vi "top level vi.vi"() -> ()   [LabVIEW 2014]
panel:
  in  "CtoF":bool
  out "Smallest":dbl
  out "greatest":dbl
  out "average value":dbl
  in  "WS":bool
  in  "stop":bool
  out "Waveform Chart":cluster{"random temp":dbl, dbl}(graph)
  # "(0~50 Celsius)"
  # "Summer"
  # "Winter"
  # "(-50~0 Celsius)"
  # "Fahrenheit"
  # "Celsius"
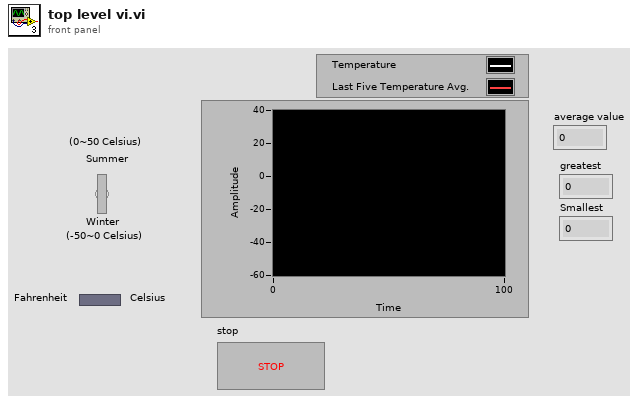
[diagram p1: front panel]
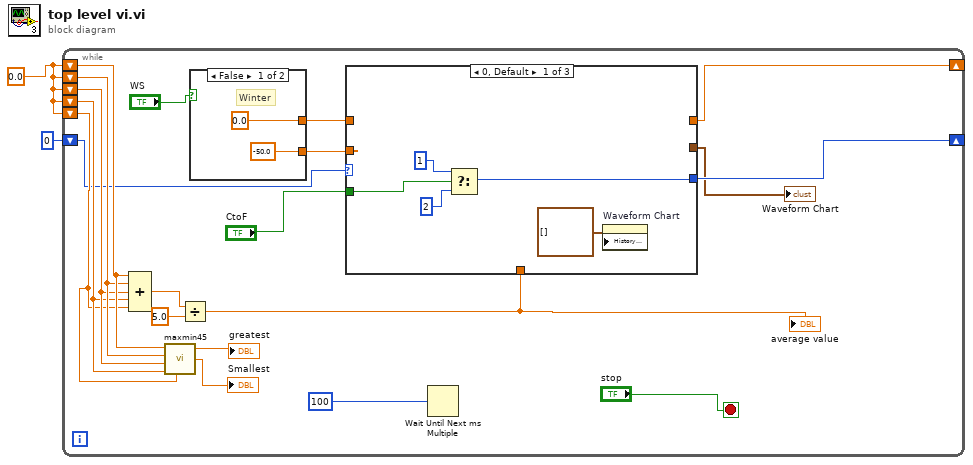
[diagram p0: block diagram]
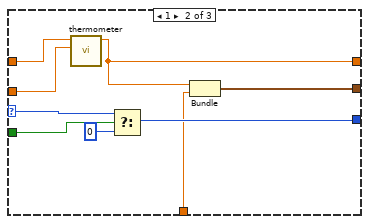
[diagram p2: hidden frame]
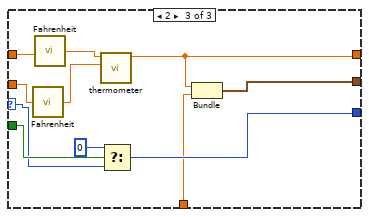
[diagram p3: hidden frame]
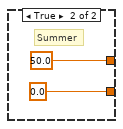
[diagram p4: hidden frame]
diagram:
  w2 = 0.0 ("random temp")
  n1 = while {
    shift-right: [w8] -> _
    shift-left: w2 -> [w17]
    shift-left: w2 -> [w16]
    shift-left: w2 -> [w14]
    shift-left: w2 -> [w15]
    shift-left: w2 -> [w13]
    shift-right: [w6] -> _
    shift-left: 0 -> [w5]
    stop <- "stop" stop-if-true
    n2 = Compound Arithmetic op=ADD(w17, w16, w15, w14, w13) -> (w19:dbl)
    n3 = call "maxmin45.vi"("Numeric"=w17, "Numeric 2"=w16, "Numeric 3"=w15, "Numeric 5"=w13, "Numeric 4"=w14) -> ("greatest"=→"greatest":dbl, "Smallest"=→"Smallest":dbl)  [unwired: 2 in]
    n4 = Divide(x=w19, y=5.0) -> (x/y=w4:dbl)
    "average value" <- w4
    n5 = case shown="False" "WS" {
      tunnel: [0.0 ("Upper Bound") 50.0 ("Upper Bound")] -> w9
      tunnel: [-50.0 ("Lower Bound") 0.0 ("Lower Bound")] -> w10
      frame False {
        # "Winter"
      }
      frame True {
        # "Summer"
      }
    }
    n6 = case shown="0, Default" w5 {
      selector: w5 -> [_ w32 w41]
      tunnel: w10 -> [_ w35 w46]
      tunnel: w9 -> [_ w36 w47]
      tunnel: [_ w31 w37] -> w8
      tunnel: "CtoF" -> [w27 w34 w43]
      tunnel: [w26 w33 w42] -> w6
      tunnel: w4 -> [_ w30 w38]
      tunnel: [_ w29 w39] -> w3
      frame 0, Default {
        n7 = Select(t=1 ("f"), s=w27, f=2) -> (s? t:f=w26:i32)
        n8 = property on="Waveform Chart" class="WFChart (strict)"("History Data"=cluster{"random temp":dbl, dbl}[] []) -> ()  [unwired: 2 in, 2 out]
      }
      frame 1 {
        n9 = call "thermometer.vi"("Lower Bound"=w35, "Upper Bound"=w36) -> ("random temp"=w31:dbl)  [unwired: 8 in, 1 out]
        n10 = Select(t=w32, s=w34, f=0) -> (s? t:f=w33:i32)
        n11 = Bundle("random temp"=w31, w30) -> (w29:cluster{"random temp":dbl, dbl})  [unwired: 1 in]
      }
      frame 2 {
        n12 = call "Fahrenheit.vi"("Celsius temperature"=w46) -> ("Fahrenheit temperature"=w44:dbl)  [unwired: 4 in]
        n13 = call "Fahrenheit.vi"("Celsius temperature"=w47) -> ("Fahrenheit temperature"=w45:dbl)  [unwired: 4 in]
        n14 = call "thermometer.vi"("Lower Bound"=w44, "Upper Bound"=w45) -> ("random temp"=w37:dbl)  [unwired: 8 in, 1 out]
        n15 = Select(t=0, s=w43, f=w41) -> (s? t:f=w42:i32)
        n16 = Bundle("random temp"=w37, w38) -> (w39:cluster{"random temp":dbl, dbl})  [unwired: 1 in]
      }
    }
    "Waveform Chart" <- w3
    n17 = Wait Until Next ms Multiple(millisecond multiple=u32 100) -> ()  [unwired: 1 out]
  }
